vi "FGV T90 Zustand.vi"(6 "Aktion":T2, 10 "Zustand":T1, 11 "T90 aktiv?":bool) -> (2 "Zustand":T1, 3 "T90 aktiv?":bool)   [LabVIEW 2020, in "T90.lvlib"]
uses:
  T90.lvlib
  Aktion FGV T90 Zustand.ctl
  Aktion Zustandsautomat.ctl
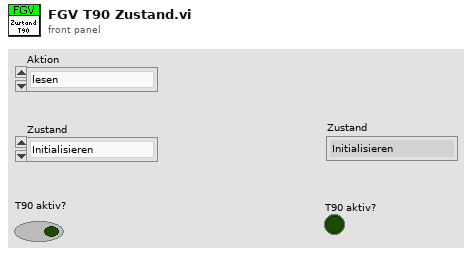
[diagram p1: front panel]
types:
  T1 = typedef "T90.lvlib/Aktion Zustandsautomat.ctl" = enum16{"Initialisieren", "Warten", "Gas aufschalten", "Volle Konzentration 1", "Berechnen", "Prüfung starten", "Prüfung", "Prüfung beenden", "keine Funktion"}
  T2 = typedef "T90.lvlib/Aktion FGV T90 Zustand.ctl" = enum16{"lesen", "T90 aktiv?", "Zustand"}
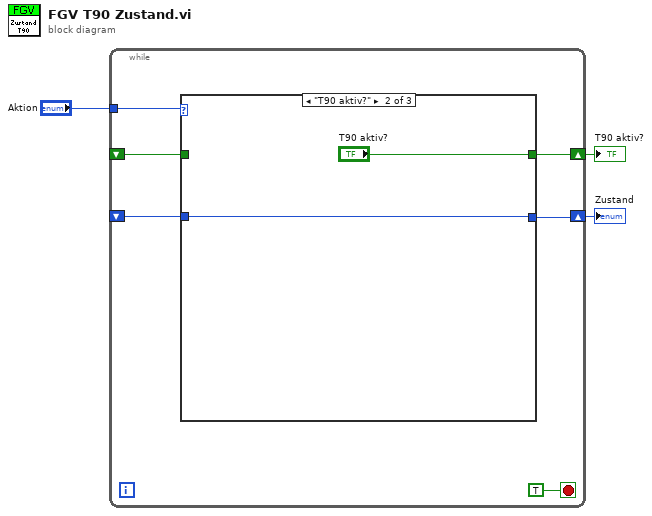
[diagram p0: block diagram]
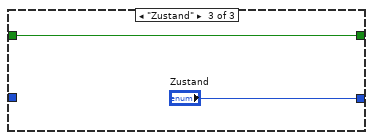
[diagram p3: hidden frame]
diagram:
  n1 = while {
    tunnel: "Aktion" -> [w8]
    shift-right: [w7] -> w2
    shift-left: _ -> [w6]
    shift-right: [w5] -> w1
    shift-left: _ -> [w4]
    stop <- TRUE stop-if-true
    n2 = case shown="\"T90 aktiv?\"" w8 {
      tunnel: [w11 "T90 aktiv?" w14] -> w7
      tunnel: w6 -> [w11 _ w14]
      tunnel: [w10 w12 "Zustand"] -> w5
      tunnel: w4 -> [w10 w12 _]
      frame "lesen", Default {
      }
      frame "T90 aktiv?" {
      }
      frame "Zustand" {
      }
    }
  }
  "T90 aktiv?" <- w2
  "Zustand" <- w1
